vi "Main.vi"() -> ()   [LabVIEW 2017]
uses:
  stateCtrl.ctl
  <vilib>/vision/driver/IMAQdx.llb/IMAQdx Camera Control Mode.ctl
  <resource>/objmgr/imaqdx.rc
  <vilib>/userdefined/High Color/IMAQdx.ctl
panel:
  out "Actual Exposure Time":dbl
  in  "Halt measurement":bool
  in  "Reset spatial\nfreqs":bool
  in  "Run":bool
  in  "stop":bool
  out "Last measurement":timestamp
  out "Measurement in progress":bool
  in  "Measurement interval (s)":dbl
  in  "Number of measurements":dbl=1.0
  in  "Current Measurement number":dbl
  in  "sampleName":string
  in  "savePath":path=path "C:/Users/Roblyer-Admin/Documents/openSFDI/Data"
  out "Current Image Index":i16
  in  "Delay":u32=200
  out "Total Images/wv":dbl
  out "numProfilometry_Images/wv":i32
  out "NumSFDI_images/wv":i32
  out "ImageMatrix":u8[][][](array[numeric])
  in  "Manual\nControl":bool
  out "Colormap":u32[](array[numeric])
  out "Arduino Session":refnum<visa-resource-name>
  in  "error":errorcluster
  out "Camera Session":T1 caption="Session Out"
  out "LED state":bool[](array[boolean])
  in  "Arduino Port":refnum<visa-resource-name>
  out "Image Array":T2[](array[plugin-control])
  in  "Prof. Spatial \nFreq (cycs)":dbl[](array[numeric])
  in  "SFDI Spatial \nFreq (cycs)":dbl[](array[numeric])
  in  "Camera Name":refnum<k21> caption="IMAQdx Session"
  in  "LED\nManual Control":enum16{"Off", "660 nm", "735 nm", "850 nm"}(ring)
  in  "Profilometry Wavelength":enum16{"None", "660 nm", "735 nm", "850 nm"}(ring)=enum."660 nm"
  in  "Dark?":bool
  in  "SFDI?":bool
  in  "Profilometry?":bool
  in  "Exposure Times (ms)":dbl[](array[numeric])=[100.0, 100.0, 100.0, 100.0]
  in  "SFDI wavelengths to use":bool[](array[boolean])
  # "660"
  # "735"
  # "850"
  # "730"
  # "865"
  # "970"
  # "660"
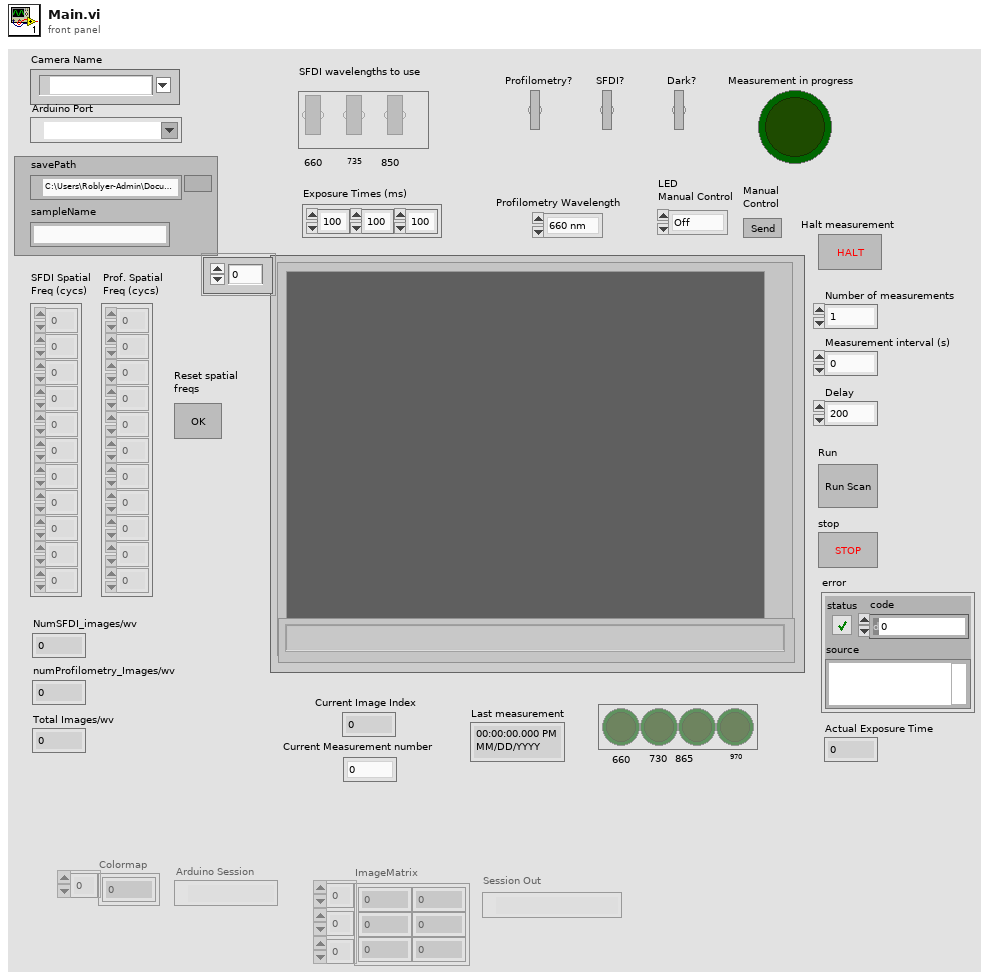
[diagram p1: front panel]
types:
  T1 = typedef "IMAQdx.ctl" = refnum<k21>
  T2 = typedef "IMAQ Image.ctl" = refnum<image>
  T3 = typedef "stateCtrl.ctl" = enum16{"Init", "Wait", "Setup Scan", "Setup Camera", "Run Scan", "Run Profilometry", "Save", "Shutdown", "Run Dark"}
  T4 = enum32{"Invalid", "Standard", "Closed", "Hidden", "Minimized", "Maximized"}
  T5 = typedef "NI_Vision_Acquisition_Software.lvlib/IMAQdx Camera Control Mode.ctl" = enum32{"Controller", "Listener"}
  T6 = cluster{"Left":i32, "Top":i32, "Right":i32, "Bottom":i32}
  T7 = typedef "Image Type" = u32
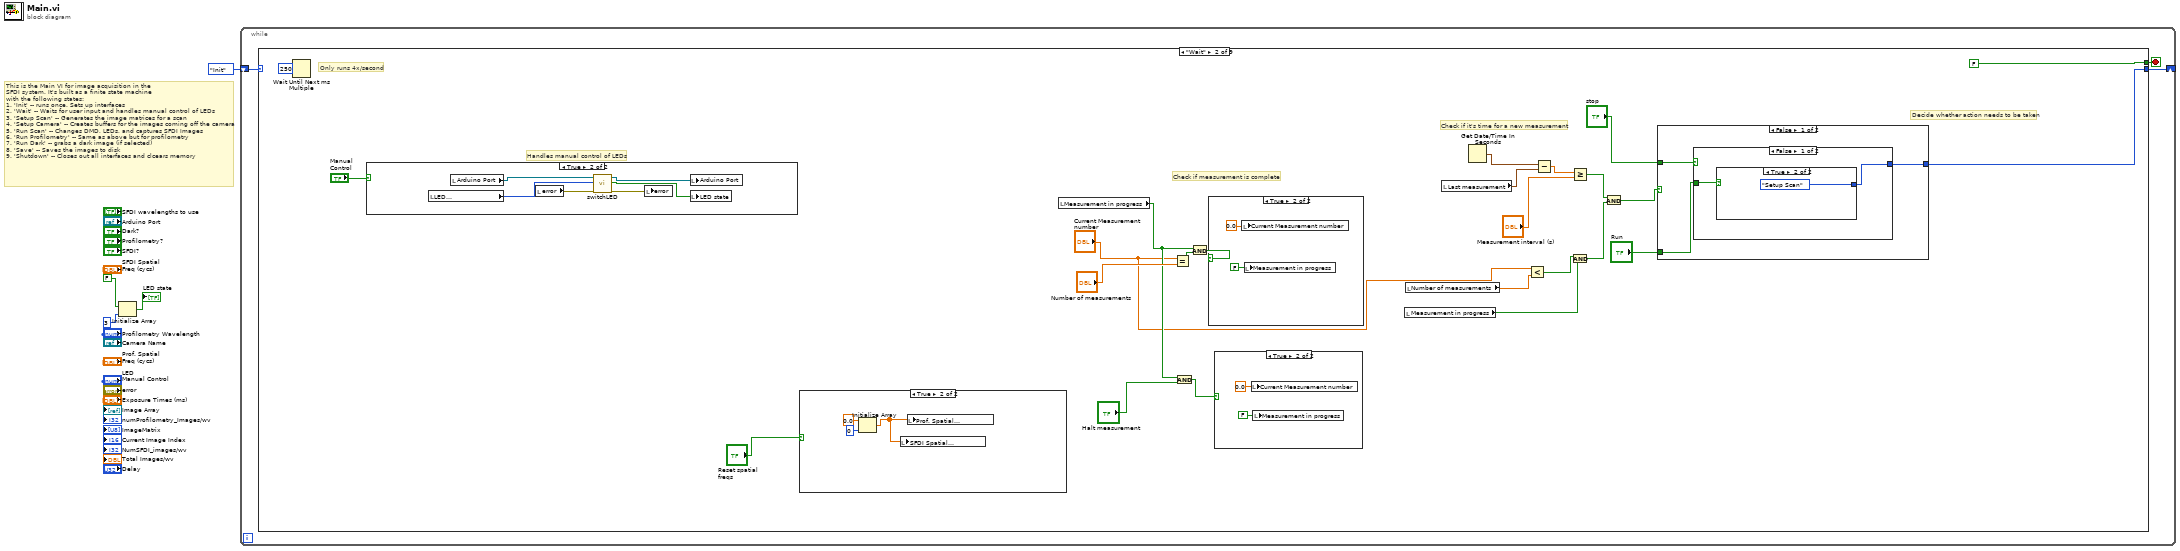
[diagram p0: block diagram]
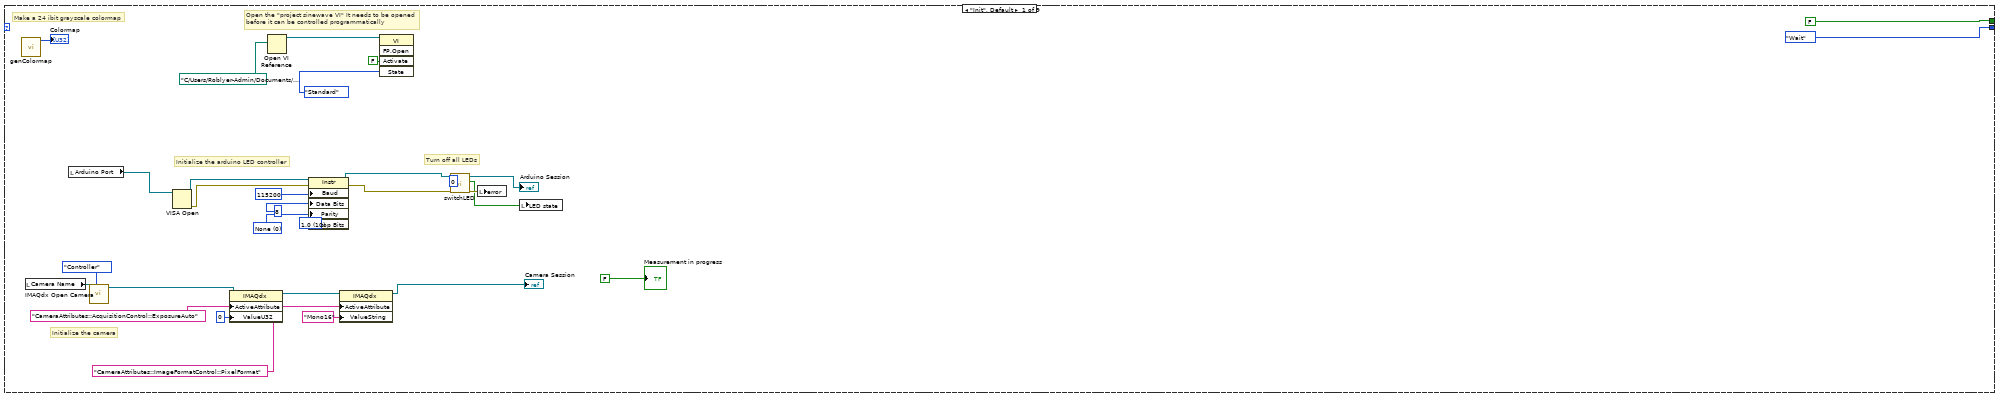
[diagram p2: hidden frame]
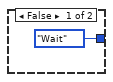
[diagram p5: hidden frame]
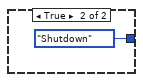
[diagram p6: hidden frame]
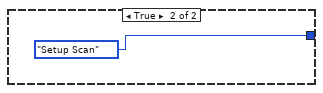
[diagram p7: hidden frame]
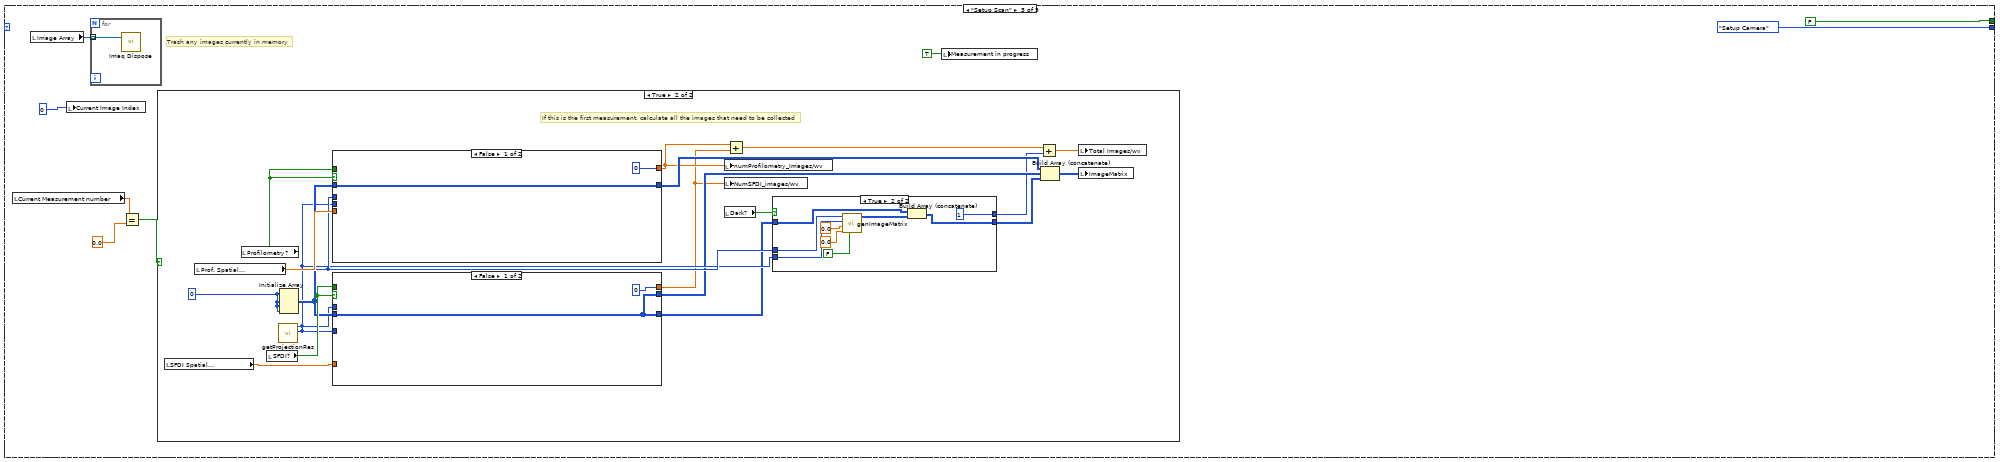
[diagram p10: hidden frame]
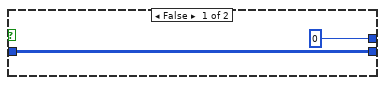
[diagram p12: hidden frame]
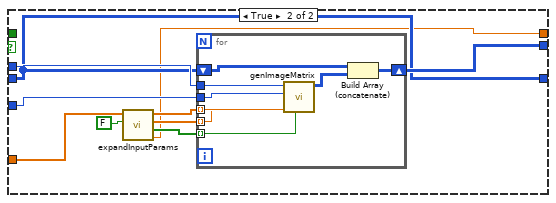
[diagram p13: hidden frame]
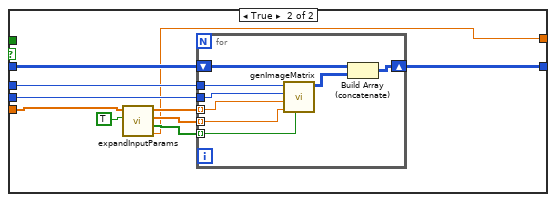
[diagram p14: hidden frame]
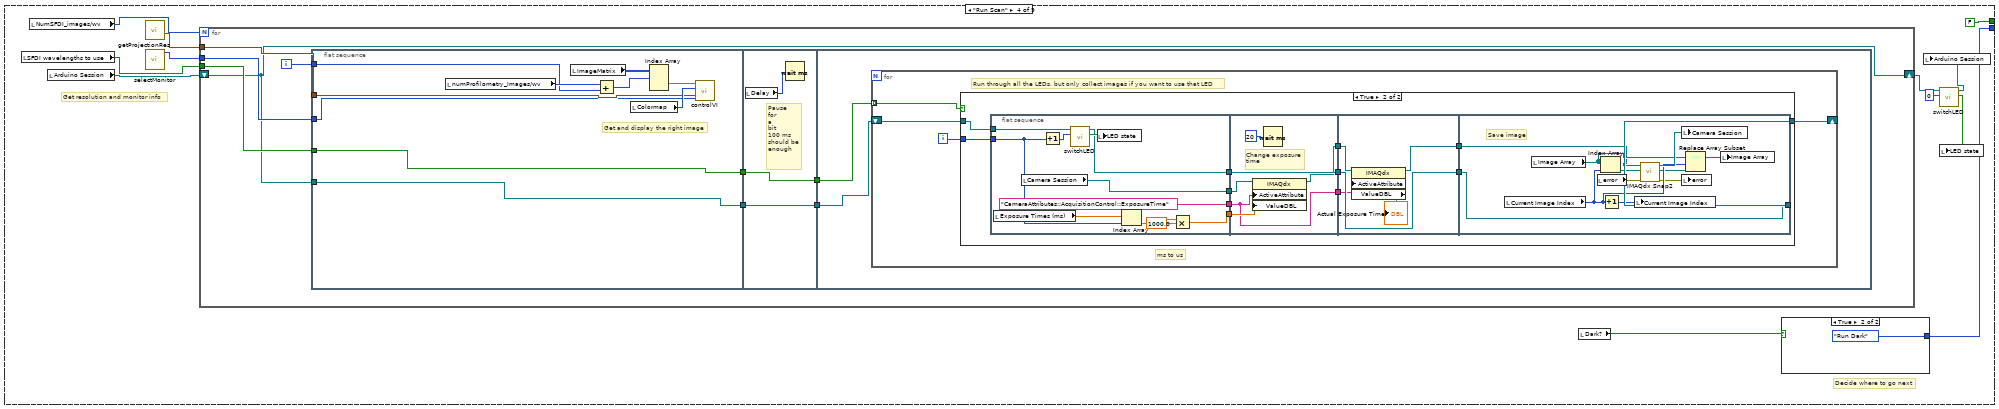
[diagram p15: hidden frame]
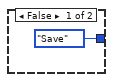
[diagram p16: hidden frame]
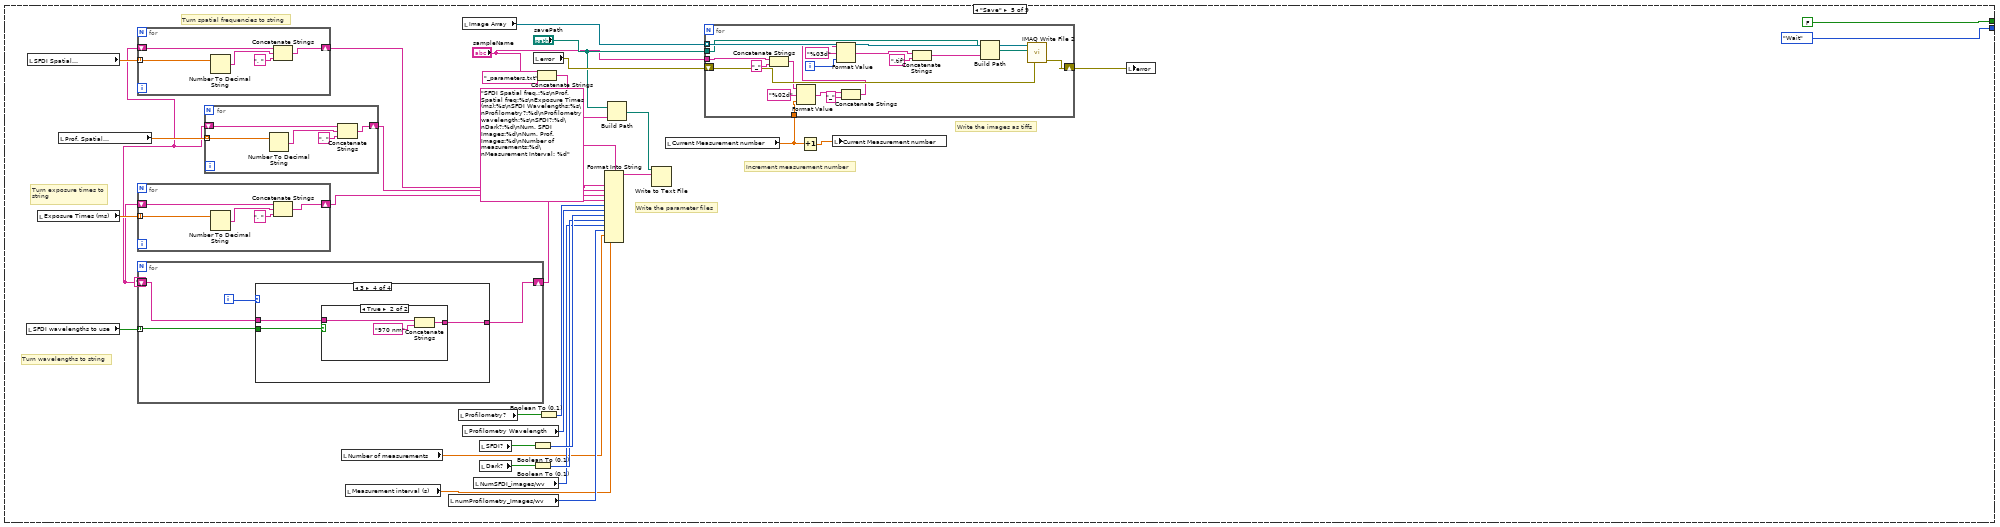
[diagram p18: hidden frame]
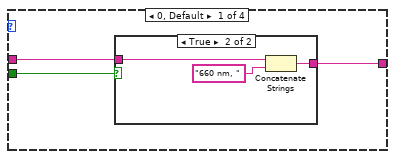
[diagram p19: hidden frame]
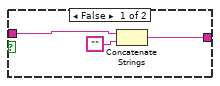
[diagram p20: hidden frame]
diagram:
  # "This is the Main VI for image acquisition in the\nSFDI system. It's built as a finite state machine\nwith the following states:\n1. 'Init' -- runs once. Sets up interfaces\n2. 'Wait' -- Waits for user input and handles manual control of LEDs\n3. 'Setup Scan' -- Generates the image matrices for a scan\n4. 'Setup Camera' -- Creates buffers for the images coming off the camera\n5. 'Run Scan' -- Changes DMD, LEDs, and captures SFDI Images\n6. 'Run Profilometry' -- Same as above but for profilometry\n7. 'Run Dark' -- grabs a dark image (if selected)\n8. 'Save' -- Saves the images to disk\n9. 'Shutdown' -- Closes out all interfaces and clcears memory"
  n1 = Initialize Array(FALSE, 3 ("dimension size")) -> (→"LED state":bool[])
  n2 = while {
    shift-right: [w5] -> _
    shift-left: stateCtrl."Init" -> [w7]
    stop <- w6 stop-if-true
    n3 = case shown="\"Wait\"" w7 {
      tunnel: [stateCtrl."Wait" w60 stateCtrl."Setup Camera" w169 stateCtrl."Wait" stateCtrl."Wait" w372 w425 stateCtrl."Save"] -> w5
      tunnel: [FALSE FALSE FALSE FALSE FALSE TRUE FALSE FALSE FALSE] -> w6
      frame "Init", Default {
        w30 = u16 10 items=["1.0"=10, "1.5"=15, "2.0"=20] ("Serial Settings:Stop Bits")
        w31 = u16 0 items=["None", "Odd", "Even", "Mark", "Space"] ("Serial Settings:Parity")
        # "Turn off all LEDs"
        # "Initialize the arduino LED controller"
        # "Initialize the camera"
        # "Open the \"project sinewave VI\" It needs to be opened \nbefore it can be controlled programmatically"
        # "Make a 24 ibit grayscale colormap"
        n4 = call "genColormap.vi"() -> ("Colormap"=→"Colormap":u32[])  [unwired: 11 in]
        n5 = local read "Camera Name"() -> (w37:refnum<k21>)
        n6 = local read "Arduino Port"() -> (w35:refnum<visa-resource-name>)
        n7 = call <vilib>:"IMAQdx Open Camera.vi"("Camera Control Mode"=IMAQdx_Camera_Control_Mode."Controller", "Session In"=w37) -> ("Session Out"=w14:T1)  [unwired: 1 in, 8 out]
        n8 = VISA Open(VISA resource name=w35) -> (VISA resource name=w34:refnum<visa-resource-name>, error out=w29:errorcluster)  [unwired: 4 in]
        n9 = property class="IMAQdx"(reference=w14, "ActiveAttribute"="CameraAttributes::AcquisitionControl::ExposureAuto", "ValueU32"=u32 0) -> (reference out=w11:T1)  [unwired: 1 in, 1 out]
        n10 = Open VI Reference(vi path=path "C:/Users/Roblyer-Admin/Documents/openSFDI/openSFDI_software/projectSinewave.vi") -> (vi reference=w27:refnum<vi>)  [unwired: 5 in, 1 out]
        n11 = property class="Instr"(reference=w34, error in=w29, "Baud"=u32 115200 ("Serial Settings:Baud Rate"), "Data Bits"=u16 8 ("Serial Settings:Data Bits"), "Parity"=w31, "Stop Bits"=w30) -> (reference out=w23:refnum<visa-resource-name>, error out=w21:errorcluster)
        n12 = property class="IMAQdx"(reference=w11, "ActiveAttribute"="CameraAttributes::ImageFormatControl::PixelFormat", "ValueString"="Mono16") -> (reference out=→"Camera Session":T1)  [unwired: 1 in, 1 out]
        n13 = invoke class="VI" method="FP.Open"(reference=w27, "Activate"=FALSE ("Activate?"), "State"=T4."Standard") -> ()  [unwired: 2 in, 5 out]
        n14 = call "switchLED.vi"("error in (no error)"=w21, "Which LED"=u8 0, "Arduino session"=w23) -> ("error out"=w19:errorcluster, "LED vector"=w17:bool[], "Arduino session"=→"Arduino Session":refnum<visa-resource-name>)  [unwired: 6 in]
        n15 = local write "error"(w19) -> ()
        n16 = local write "LED state"(w17) -> ()
        "Measurement in progress" <- FALSE ("Measurement in progress")
      }
      frame "Wait" {
        # "Decide whether action needs to be taken"
        # "Check if it's time for a new measurement"
        # "Check if measurement is complete"
        # "Handles manual control of LEDs"
        # "Only runs 4x/second"
        n17 = Wait Until Next ms Multiple(millisecond multiple=u32 250 ("milliseconds to wait")) -> ()  [unwired: 1 out]
        n18 = case shown="True" "Manual\nControl" {
          frame False {
          }
          frame True {
            n19 = local read "LED\nManual Control"() -> (w83:enum16{"Off", "660 nm", "735 nm", "850 nm"})
            n20 = local read "Arduino Port"() -> (w82:refnum<visa-resource-name>)
            n21 = local read "error"() -> (w81:errorcluster)
            n22 = call "switchLED.vi"("error in (no error)"=w81, "Which LED"=w83, "Arduino session"=w82) -> ("error out"=w78:errorcluster, "LED vector"=w80:bool[], "Arduino session"=w79:refnum<visa-resource-name>)  [unwired: 6 in]
            n23 = local write "error"(w78) -> ()
            n24 = local write "Arduino Port"(w79) -> ()
            n25 = local write "LED state"(w80) -> ()
          }
        }
        n26 = case shown="True" "Reset spatial\nfreqs" {
          frame False {
          }
          frame True {
            n27 = Initialize Array(0.0 ("element"), 0 ("dimension size")) -> (w64:dbl[])
            n28 = local write "SFDI Spatial \nFreq (cycs)"(w64) -> ()
            n29 = local write "Prof. Spatial \nFreq (cycs)"(w64) -> ()
          }
        }
        n30 = local read "Measurement in progress"() -> (w41:bool)
        n31 = Equal?(x="Current Measurement number", y="Number of measurements") -> (x = y?=w52:bool)
        n32 = And(x=w41, y="Halt measurement") -> (x .and. y?=w43:bool)
        n33 = And(x=w41, y=w52) -> (x .and. y?=w51:bool)
        n34 = case shown="True" w51 {
          frame False {
          }
          frame True {
            n35 = local write "Current Measurement number"(0.0 ("Current Measurement number")) -> ()
            n36 = local write "Measurement in progress"(FALSE ("Measurement in progress")) -> ()
          }
        }
        n37 = case shown="True" w43 {
          frame False {
          }
          frame True {
            n38 = local write "Current Measurement number"(0.0 ("Current Measurement number")) -> ()
            n39 = local write "Measurement in progress"(FALSE ("Measurement in progress")) -> ()
          }
        }
        n40 = local read "Measurement in progress"() -> (w48:bool)
        n41 = local read "Number of measurements"() -> (w50:dbl)
        n42 = local read "Last measurement"() -> (w56:timestamp)
        n43 = Get Date/Time In Seconds() -> (seconds since 1Jan1904=w57:timestamp)
        n44 = Less?(x="Current Measurement number", y=w50) -> (x < y?=w49:bool)
        n45 = Subtract(x=w57, y=w56) -> (x-y=w55:dbl)
        n46 = Greater Or Equal?(x=w55, y="Measurement interval (s)") -> (x >= y?=w47:bool)
        n47 = And(x=w49, y=w48) -> (x .and. y?=w46:bool)
        n48 = And(x=w47, y=w46) -> (x .and. y?=w45:bool)
        n49 = case shown="False" w45 {
          tunnel: [w69 stateCtrl."Setup Scan"] -> w60
          tunnel: "stop" -> [w68 _]
          tunnel: "Run" -> [w67 _]
          frame False {
            n50 = case shown="False" w68 {
              tunnel: [w70 stateCtrl."Shutdown"] -> w69
              tunnel: w67 -> [w71 _]
              frame False {
                n51 = case shown="True" w71 {
                  tunnel: [stateCtrl."Wait" stateCtrl."Setup Scan"] -> w70
                  frame False {
                  }
                  frame True {
                  }
                }
              }
              frame True {
              }
            }
          }
          frame True {
          }
        }
      }
      frame "Setup Scan" {
        # "Trash any images currently in memory"
        n52 = local read "Current Measurement number"() -> (w87:dbl)
        n53 = local read "Image Array"() -> (w88:T2[])
        n54 = local write "Current Image Index"(i16 0 ("Current Image Index")) -> ()
        n55 = for {
          tunnel: w88 -> [w162] mode=indexing
          n56 = call "Imaq Dispose"("Image"=w162) -> ()  [unwired: 5 in, 1 out]
        }
        n57 = Equal?(x=w87, y=0.0) -> (x = y?=w85:bool)
        n58 = case shown="True" w85 {
          frame False {
          }
          frame True {
            w105 = 0
            # "If this is the first measurement, calculate all the images that need to be collected"
            n59 = local read "SFDI Spatial \nFreq (cycs)"() -> (w106:dbl[])
            n60 = local read "Prof. Spatial \nFreq (cycs)"() -> (w108:dbl[])
            n61 = local read "Profilometry?"() -> (w109:bool)
            n62 = local read "SFDI?"() -> (w107:bool)
            n63 = call "getProjectionRes.vi"() -> ("YRes"=w102:i32, "XRes"=w103:i32)  [unwired: 9 in, 1 out]
            n64 = Initialize Array(w105, w105, w105, w105) -> (w104:i32[][][])
            n65 = case shown="False" w109 {
              tunnel: w103 -> [_ w150]
              tunnel: w102 -> [_ w149]
              tunnel: w109 -> [_ _]
              tunnel: w108 -> [_ w148]
              tunnel: w104 -> [w143 w147]
              tunnel: [w143 w145] -> w101
              tunnel: [0 w144] -> w96
              frame False {
              }
              frame True {
                n66 = call "expandInputParams.vi"("Profilometry?"=TRUE, "Frequencies"=w148) -> ("Number Images"=w144:dbl, "Orientation Vector"=w153:bool[], "Phase Vector"=w152:dbl[], "Frequency Vector"=w151:dbl[])  [unwired: 6 in]
                n67 = for {
                  tunnel: w153 -> [w161] mode=indexing
                  tunnel: w152 -> [w160] mode=indexing
                  tunnel: w151 -> [w159] mode=indexing
                  tunnel: w150 -> [w158]
                  tunnel: w149 -> [w157]
                  shift-right: [w155] -> w145
                  shift-left: w147 -> [w154]
                  n68 = call "genImageMatrix.vi"("Orientation"=w161, "Phase"=w160, "Cycles"=w159, "Y resolution"=w157, "X Resolution"=w158) -> ("Scan Image"=w156:u8[][])  [unwired: 5 in, 1 out]
                  n69 = Build Array (concatenate)(w154, w156) -> (w155:i32[][][])
                }
              }
            }
            n70 = case shown="False" w107 {
              tunnel: w107 -> [_ _]
              tunnel: w106 -> [_ w133]
              tunnel: w104 -> [w123 w125]
              tunnel: w103 -> [_ w131]
              tunnel: w102 -> [_ w130]
              tunnel: [w123 w126] -> w100
              tunnel: [w123 w125] -> w98
              tunnel: [0 w124] -> w95
              frame False {
              }
              frame True {
                n71 = call "expandInputParams.vi"("Profilometry?"=FALSE, "Frequencies"=w133) -> ("Number Images"=w124:dbl, "Orientation Vector"=w127:bool[], "Phase Vector"=w128:dbl[], "Frequency Vector"=w129:dbl[])  [unwired: 6 in]
                n72 = for {
                  shift-right: [w140] -> w126
                  shift-left: w125 -> [w139]
                  tunnel: w131 -> [w138]
                  tunnel: w130 -> [w137]
                  tunnel: w129 -> [w136] mode=indexing
                  tunnel: w128 -> [w135] mode=indexing
                  tunnel: w127 -> [w134] mode=indexing
                  n73 = call "genImageMatrix.vi"("Orientation"=w134, "Phase"=w135, "Cycles"=w136, "Y resolution"=w137, "X Resolution"=w138) -> ("Scan Image"=w141:u8[][])  [unwired: 5 in, 1 out]
                  n74 = Build Array (concatenate)(w139, w141) -> (w140:i32[][][])
                }
              }
            }
            n75 = local write "numProfilometry_Images/wv"(w96) -> ()
            n76 = local write "NumSFDI_images/wv"(w95) -> ()
            n77 = local read "Dark?"() -> (w110:bool)
            n78 = Add(x=w96, y=w95) -> (x+y=w94:dbl)
            n79 = case shown="True" w110 {
              tunnel: w103 -> [_ w121]
              tunnel: w102 -> [_ w120]
              tunnel: [w112 w114] -> w99
              tunnel: w98 -> [w112 w116]
              tunnel: [0 1] -> w93
              frame False {
              }
              frame True {
                n80 = call "genImageMatrix.vi"("Orientation"=FALSE, "Phase"=0.0, "Cycles"=0.0, "Y resolution"=w120, "X Resolution"=w121) -> ("Scan Image"=w115:u8[][])  [unwired: 5 in, 1 out]
                n81 = Build Array (concatenate)(w116, w115) -> (w114:i32[][][])
              }
            }
            n82 = Add(x=w94, y=w93) -> (x+y=w92:dbl)
            n83 = Build Array (concatenate)(w101, w100, w99) -> (w97:i32[][][])
            n84 = local write "Total Images/wv"(w92) -> ()
            n85 = local write "ImageMatrix"(w97) -> ()
          }
        }
        n86 = local write "Measurement in progress"(TRUE) -> ()
      }
      frame "Run Scan" {
        # "Decide where to go next"
        # "Get resolution and monitor info"
        n87 = local read "SFDI wavelengths to use"() -> (w170:bool[])
        n88 = local read "NumSFDI_images/wv"() -> (w168:i32)
        n89 = local read "Arduino Session"() -> (w171:refnum<visa-resource-name>)
        n90 = call "getProjectionRes.vi"() -> ("projBounds"=w173:T6)  [unwired: 9 in, 2 out]
        n91 = call "selectMonitor.vi"() -> ("monitor to use"=w172:i32)  [unwired: 11 in]
        n92 = for {
          N: w168 -> [_]
          tunnel: w173 -> [w184]
          tunnel: w172 -> [w183]
          tunnel: w170 -> [w180]
          shift-right: [w177] -> w166
          shift-left: w171 -> [w177]
          i -> [w185]
          n93 = flat-sequence {
            tunnel: w185 -> [w194]
            tunnel: w184 -> [w189]
            tunnel: w183 -> [w188]
            tunnel: [w187] -> w181
            tunnel: w180 -> [w187]
            tunnel: [w186] -> w178
            tunnel: w177 -> [w186]
            tunnel: [w198] -> w182
            tunnel: w181 -> [w198]
            tunnel: [w197] -> w179
            tunnel: w178 -> [w197]
            tunnel: w182 -> [w200]
            tunnel: w179 -> [w199]
            frame #0 {
              # "Get and display the right image"
              n94 = local read "numProfilometry_Images/wv"() -> (w195:i32)
              n95 = local read "ImageMatrix"() -> (w193:u8[][][])
              n96 = Add(x=w195, y=w194) -> (x+y=w192:i32)
              n97 = local read "Colormap"() -> (w190:u32[])
              n98 = Index Array(array=w193, index (dim 0)=w192) -> (element=w191:u8[][])  [unwired: 2 in]
              n99 = call "controlVI.vi"("monitorToUse"=w188, "Front Panel Window:Window Bounds"=w189, "colors"=w190, "8-bit pixmap"=w191) -> ()  [unwired: 7 in, 1 out]
            }
            frame #1 {
              # "Pause\nfor\na\nbit\n100 ms\nshould be\nenough"
              n100 = local read "Delay"() -> (w196:u32)
              n101 = Wait (ms)(milliseconds to wait=w196) -> ()  [unwired: 1 out]
            }
            frame #2 {
              n102 = for {
                shift-right: [w202] -> _
                shift-left: w199 -> [w203]
                tunnel: w200 -> [w201] mode=indexing
                i -> [w204]
                # "ms to us"
                # "Run through all the LEDs, but only collect images if you want to use that LED"
                n103 = case shown="True" w201 {
                  tunnel: w204 -> [_ w217]
                  tunnel: w203 -> [w205 w216]
                  tunnel: [w205 w215] -> w202
                  frame False {
                  }
                  frame True {
                    n104 = flat-sequence {
                      tunnel: w217 -> [w221]
                      tunnel: w216 -> [w227]
                      tunnel: [w225] -> w214
                      tunnel: [w224] -> w213
                      tunnel: ["CameraAttributes::AcquisitionControl::ExposureTime"] -> w212
                      tunnel: [w218] -> w211
                      tunnel: [w233] -> w210
                      tunnel: w214 -> [w233]
                      tunnel: [w231] -> w208
                      tunnel: w213 -> [w232]
                      tunnel: w212 -> [w229]
                      tunnel: w211 -> [w230]
                      tunnel: [w229] -> w206
                      tunnel: w210 -> [w237]
                      tunnel: [w237] -> w209
                      tunnel: w208 -> [w239]
                      tunnel: [w238] -> w207
                      tunnel: w206 -> [w235]
                      tunnel: [w243] -> w215
                      tunnel: w209 -> [w243]
                      tunnel: w207 -> [w240]
                      frame #0 {
                        n105 = local read "Exposure Times (ms)"() -> (w222:dbl[])
                        n106 = local read "Camera Session"() -> (w224:T1)
                        n107 = Increment(x=w221) -> (x+1=w228:i32)
                        n108 = call "switchLED.vi"("Which LED"=w228, "Arduino session"=w227) -> ("LED vector"=w226:bool[], "Arduino session"=w225:refnum<visa-resource-name>)  [unwired: 7 in, 1 out]
                        n109 = local write "LED state"(w226) -> ()
                        n110 = Index Array(array=w222, index=w221) -> (element=w220:dbl)
                        n111 = Multiply(x=w220, y=1000.0) -> (x*y=w218:dbl)
                      }
                      frame #1 {
                        # "Change exposure\ntime"
                        n112 = property class="IMAQdx"(reference=w232, "ActiveAttribute"=w229, "ValueDBL"=w230) -> (reference out=w231:T1)  [unwired: 1 in, 1 out]
                        n113 = Wait (ms)(milliseconds to wait=u32 20) -> ()  [unwired: 1 out]
                      }
                      frame #2 {
                        n114 = property class="IMAQdx"(reference=w239, "ActiveAttribute"=w235) -> (reference out=w238:T1, "ValueDBL"=→"Actual Exposure Time")  [unwired: 1 in, 1 out]
                      }
                      frame #3 {
                        # "Save image"
                        n115 = local read "Current Image Index"() -> (w246:i16)
                        n116 = local read "Image Array"() -> (w247:T2[])
                        n117 = local read "error"() -> (w242:errorcluster)
                        n118 = Index Array(array=w247, index=w246) -> (element=w249:T2)
                        n119 = Increment(x=w246) -> (x+1=w248:i16)
                        n120 = local write "Current Image Index"(w248) -> ()
                        n121 = call <vilib>:"IMAQdx Snap2.vi"("error in"=w242, "Image In"=w249, "Session In"=w240) -> ("error out"=w241:errorcluster, "Image Out"=w245:T2, "Session Out"=w250:T1)  [unwired: 6 in]
                        n122 = local write "Camera Session"(w250) -> ()
                        n123 = local write "error"(w241) -> ()
                        n124 = Replace Array Subset(array=w247, new element=w245, index=w246) -> (w244:T2[])
                        n125 = local write "Image Array"(w244) -> ()
                      }
                    }
                  }
                }
              }
            }
          }
        }
        n126 = local read "Dark?"() -> (w167:bool)
        n127 = case shown="True" w167 {
          tunnel: [stateCtrl."Save" stateCtrl."Run Dark"] -> w169
          frame False {
          }
          frame True {
          }
        }
        n128 = call "switchLED.vi"("Which LED"=u8 0, "Arduino session"=w166) -> ("LED vector"=w164:bool[], "Arduino session"=w163:refnum<visa-resource-name>)  [unwired: 7 in, 1 out]
        n129 = local write "Arduino Session"(w163) -> ()
        n130 = local write "LED state"(w164) -> ()
      }
      frame "Save" {
        w257 = ""
        # "Increment measurement number"
        # "Write the images as tiffs"
        # "Write the parameter files"
        # "Turn wavelengths to string"
        # "Turn exposure times to\nstring"
        # "Turn spatial frequencies to string"
        n131 = local read "SFDI wavelengths to use"() -> (w255:bool[])
        n132 = local read "SFDI Spatial \nFreq (cycs)"() -> (w276:dbl[])
        n133 = local read "Exposure Times (ms)"() -> (w274:dbl[])
        n134 = local read "Prof. Spatial \nFreq (cycs)"() -> (w275:dbl[])
        n135 = for {
          tunnel: w276 -> [w339] mode=indexing
          shift-right: [w336] -> w273
          shift-left: w257 -> [w335]
          n136 = Number To Decimal String(number=w339) -> (decimal integer string=w337:string)  [unwired: 1 in]
          n137 = Concatenate Strings(w335, w337, ", ") -> (w336:string)
        }
        n138 = for {
          tunnel: w274 -> [w329] mode=indexing
          shift-right: [w326] -> w271
          shift-left: w257 -> [w325]
          n139 = Number To Decimal String(number=w329) -> (decimal integer string=w327:string)  [unwired: 1 in]
          n140 = Concatenate Strings(w325, w327, ", ") -> (w326:string)
        }
        n141 = for {
          shift-right: [w286] -> w270
          shift-left: w257 -> [w285]
          tunnel: w255 -> [w287] mode=indexing
          i -> [w288]
          n142 = case shown="3" w288 {
            tunnel: w287 -> [w291 w300 w309 w318]
            tunnel: [w290 w299 w308 w316] -> w286
            tunnel: w285 -> [w289 w298 w307 w317]
            frame 0, Default {
              n143 = case shown="True" w291 {
                tunnel: [w294 w295] -> w290
                tunnel: w289 -> [w293 w297]
                frame False {
                  n144 = Concatenate Strings(w293, "") -> (w294:string)
                }
                frame True {
                  n145 = Concatenate Strings(w297, "660 nm, ") -> (w295:string)
                }
              }
            }
            frame 1 {
              n146 = case shown="True" w300 {
                tunnel: [w301 w304] -> w299
                tunnel: w298 -> [w303 w306]
                frame False {
                  n147 = Concatenate Strings(w303, "") -> (w301:string)
                }
                frame True {
                  n148 = Concatenate Strings(w306, "730 nm, ") -> (w304:string)
                }
              }
            }
            frame 2 {
              n149 = case shown="True" w309 {
                tunnel: [w310 w313] -> w308
                tunnel: w307 -> [w312 w314]
                frame False {
                  n150 = Concatenate Strings(w312, "") -> (w310:string)
                }
                frame True {
                  n151 = Concatenate Strings(w314, "865 nm, ") -> (w313:string)
                }
              }
            }
            frame 3 {
              n152 = case shown="True" w318 {
                tunnel: w317 -> [w321 w324]
                tunnel: [w319 w322] -> w316
                frame False {
                  n153 = Concatenate Strings(w321, "") -> (w319:string)
                }
                frame True {
                  n154 = Concatenate Strings(w324, "970 nm") -> (w322:string)
                }
              }
            }
          }
        }
        n155 = for {
          tunnel: w275 -> [w334] mode=indexing
          shift-right: [w331] -> w272
          shift-left: w257 -> [w330]
          n156 = Number To Decimal String(number=w334) -> (decimal integer string=w332:string)  [unwired: 1 in]
          n157 = Concatenate Strings(w330, w332, ", ") -> (w331:string)
        }
        n158 = local read "Number of measurements"() -> (w252:dbl)
        n159 = local read "Measurement interval (s)"() -> (w251:dbl)
        n160 = local read "numProfilometry_Images/wv"() -> (w259:i32)
        n161 = local read "Profilometry?"() -> (w277:bool)
        n162 = local read "Image Array"() -> (w282:T2[])
        n163 = local read "Profilometry Wavelength"() -> (w256:enum16{"None", "660 nm", "735 nm", "850 nm"})
        n164 = local read "NumSFDI_images/wv"() -> (w260:i32)
        n165 = local read "SFDI?"() -> (w278:bool)
        n166 = local read "Dark?"() -> (w279:bool)
        n167 = Boolean To (0,1)(Boolean=w278) -> (0, 1=w268:i16)
        n168 = Boolean To (0,1)(Boolean=w279) -> (0, 1=w267:i16)
        n169 = local read "error"() -> (w281:errorcluster)
        n170 = Concatenate Strings("sampleName", "_parameters.txt" ("string")) -> (w263:string)
        n171 = Boolean To (0,1)(Boolean=w277) -> (0, 1=w269:i16)
        n172 = Format Into String(format string="SFDI Spatial freq.:%s\nProf. Spatial freq:%s\nExposure Times (ms):%s\nSFDI Wavelengths:%s\nProfilometry?:%d\nProfilometry wavelength:%s\nSFDI?:%d\nDark?:%d\nNum. SFDI Images:%d\nNum. Prof. Images:%d\nNumber of measurements:%d\nMeasurement Interval: %d", w273, w272, w271, w270, w269, w256, w268, w267, w260, w259, w252, w251) -> (resulting string=w261:string)  [unwired: 2 in, 1 out]
        n173 = Build Path(base path="savePath", name or relative path=w263) -> (appended path=w262:path)
        n174 = Write to Text File(file (use dialog)=w262, text=w261) -> ()  [unwired: 2 in, 3 out]
        n175 = local read "Current Measurement number"() -> (w253:dbl)
        n176 = for {
          tunnel: w282 -> [w357] mode=indexing
          shift-right: [w346] -> w280
          shift-left: w281 -> [w356]
          tunnel: "savePath" -> [w355]
          tunnel: "sampleName" -> [w347]
          tunnel: w253 -> [w344]
          i -> [w352]
          n177 = Concatenate Strings(w347, "_") -> (w343:string)
          n178 = Format Value(string ("")=w343, format string="%02d", value (0)=w344) -> (output string=w342:string)
          n179 = Concatenate Strings(w342, "_" ("string")) -> (w340:string)
          n180 = Format Value(string ("")=w340, format string="%03d", value (0)=w352) -> (output string=w351:string)
          n181 = Concatenate Strings(w351, ".tif" ("string")) -> (w349:string)
          n182 = Build Path(base path=w355, name or relative path=w349) -> (appended path=w348:path)
          n183 = call-poly "IMAQ Write File 2"("error in (no error)"=w356, "File Path"=w348, "Image"=w357) -> ("error out"=w346:errorcluster)  [unwired: 7 in, 1 out]
        }
        n184 = Increment(x=w253) -> (x+1=w254:dbl)
        n185 = local write "Current Measurement number"(w254) -> ()
        n186 = local write "error"(w280) -> ()
      }
      frame "Shutdown" {
        # "Stop the while loop"
        # "Turn off and close session with Arduino"
        # "Close camera"
        # "Clean up memory"
        n187 = local read "Image Array"() -> (w358:T2[])
        n188 = local read "Camera Session"() -> (w363:T1)
        n189 = for {
          tunnel: w358 -> [w368] mode=indexing
          n190 = call "Imaq Dispose"("Image"=w368) -> ()  [unwired: 5 in, 1 out]
        }
        n191 = local read "error"() -> (w362:errorcluster)
        n192 = local read "Arduino Session"() -> (w365:refnum<visa-resource-name>)
        n193 = call <vilib>:"IMAQdx Close Camera.vi"("error in"=w362, "Session In"=w363) -> ("error out"=w361:errorcluster)  [unwired: 9 out]
        n194 = call "switchLED.vi"("error in (no error)"=w361, "Which LED"=u8 0, "Arduino session"=w365) -> ("error out"=w360:errorcluster, "Arduino session"=w364:refnum<visa-resource-name>)  [unwired: 6 in, 1 out]
        n195 = VISA Close(VISA resource name=w364, error in (no error)=w360) -> ()  [unwired: 1 out]
      }
      frame "Run Profilometry" {
        # "Decide whether Dark, or SFDI needs to be done"
        # "Turn off LEDs when done"
        # "Turn on LED"
        # "Profilometry always comes before SFDI or Dark\nmeasurements"
        n196 = local read "Profilometry Wavelength"() -> (w384:enum16{"None", "660 nm", "735 nm", "850 nm"})
        n197 = local read "Arduino Session"() -> (w383:refnum<visa-resource-name>)
        n198 = local read "numProfilometry_Images/wv"() -> (w370:i32)
        n199 = local read "error"() -> (w382:errorcluster)
        n200 = call "switchLED.vi"("error in (no error)"=w382, "Which LED"=w384, "Arduino session"=w383) -> ("error out"=w377:errorcluster, "LED vector"=w381:bool[], "Arduino session"=w379:refnum<visa-resource-name>)  [unwired: 6 in]
        n201 = local write "LED state"(w381) -> ()
        n202 = for {
          N: w370 -> [_]
          shift-right: [w391] -> w378
          shift-left: w377 -> [w390]
          i -> [w394]
          # "Take an image for each profilometry pattern selected"
          n203 = flat-sequence {
            tunnel: w394 -> [w400]
            tunnel: [w395] -> w392
            tunnel: w390 -> [w395]
            tunnel: [w402] -> w393
            tunnel: w392 -> [w402]
            tunnel: w393 -> [w411]
            tunnel: [w407] -> w391
            frame #0 {
              # "Project pattern"
              n204 = local read "ImageMatrix"() -> (w401:u8[][][])
              n205 = local read "Colormap"() -> (w399:u32[])
              n206 = Index Array(array=w401, index (dim 0)=w400) -> (element=w398:u8[][])  [unwired: 2 in]
              n207 = call "getProjectionRes.vi"() -> ("projBounds"=w397:T6)  [unwired: 9 in, 2 out]
              n208 = call "selectMonitor.vi"() -> ("monitor to use"=w396:i32)  [unwired: 11 in]
              n209 = call "controlVI.vi"("monitorToUse"=w396, "Front Panel Window:Window Bounds"=w397, "colors"=w399, "8-bit pixmap"=w398) -> ()  [unwired: 7 in, 1 out]
            }
            frame #1 {
              n210 = local read "Delay"() -> (w403:u32)
              n211 = Wait (ms)(milliseconds to wait=w403) -> ()  [unwired: 1 out]
            }
            frame #2 {
              n212 = local read "Current Image Index"() -> (w405:i16)
              n213 = local read "Image Array"() -> (w409:T2[])
              n214 = local read "Camera Session"() -> (w413:T1)
              n215 = Increment(x=w405) -> (x+1=w406:i16)
              n216 = Index Array(array=w409, index=w405) -> (element=w412:T2)
              n217 = local write "Current Image Index"(w406) -> ()
              n218 = call <vilib>:"IMAQdx Snap2.vi"("error in"=w411, "Image In"=w412, "Session In"=w413) -> ("error out"=w407:errorcluster, "Image Out"=w410:T2, "Session Out"=w404:T1)  [unwired: 6 in]
              n219 = Replace Array Subset(array=w409, new element=w410, index=w405) -> (w408:T2[])
              n220 = local write "Camera Session"(w404) -> ()
              n221 = local write "Image Array"(w408) -> ()
            }
          }
        }
        n222 = call "switchLED.vi"("error in (no error)"=w378, "Which LED"=u8 0, "Arduino session"=w379) -> ("error out"=w375:errorcluster, "LED vector"=w376:bool[], "Arduino session"=w374:refnum<visa-resource-name>)  [unwired: 6 in]
        n223 = local write "error"(w375) -> ()
        n224 = local write "Arduino Session"(w374) -> ()
        n225 = local write "LED state"(w376) -> ()
        n226 = local read "SFDI?"() -> (w373:bool)
        n227 = local read "Dark?"() -> (w369:bool)
        n228 = case shown="False" w373 {
          tunnel: [w385 stateCtrl."Run Scan"] -> w372
          tunnel: w369 -> [w386 _]
          frame False {
            n229 = case shown="False" w386 {
              tunnel: [stateCtrl."Save" stateCtrl."Run Dark"] -> w385
              frame False {
              }
              frame True {
              }
            }
          }
          frame True {
          }
        }
      }
      frame "Setup Camera" {
        # "Decide where to go next"
        # "Save start time"
        # "Calculate total number of images to collect"
        # "Do camera stuff here"
        n230 = local read "SFDI wavelengths to use"() -> (w424:bool[])
        n231 = Boolean To (0,1)(Boolean=w424) -> (0, 1=w423:i16[])
        n232 = local read "NumSFDI_images/wv"() -> (w421:i32)
        n233 = local read "numProfilometry_Images/wv"() -> (w419:i32)
        n234 = Add Array Elements(numeric array=w423) -> (sum=w422:i16)
        n235 = Multiply(x=w422, y=w421) -> (x*y=w420:i32)
        n236 = Add(x=w420, y=w419) -> (x+y=w416:i32)
        n237 = local read "Dark?"() -> (w417:bool)
        n238 = case shown="False" w417 {
          tunnel: w416 -> [w430 w432]
          tunnel: [w430 w431] -> w415
          frame False {
          }
          frame True {
            n239 = Increment(x=w432) -> (x+1=w431:i32)
          }
        }
        n240 = local read "error"() -> (w429:errorcluster)
        n241 = for {
          N: w415 -> [_]
          tunnel: w429 -> [w448]
          tunnel: [w447] -> w427 mode=indexing
          tunnel: [w446] -> w428
          i -> [w445]
          w442 = T7 7 items=["Grayscale (U8)", "Grayscale (I16)", "Grayscale (SGL)", "Complex (CSG)", "RGB (U32)", "HSL (U32)", "RGB (U64)", "Grayscale (U16)"] ("Image Type")
          # "Reserve memory for images"
          n242 = Format Into String(format string="image%d" ("Image Name"), w445) -> (resulting string=w444:string)  [unwired: 2 in, 1 out]
          n243 = call "IMAQ Create"("Image Name"=w444, "Image Type"=w442, "error in (no error)"=w448) -> ("New Image"=w447:T2, "error out"=w446:errorcluster)  [unwired: 1 in, 1 out]
        }
        n244 = Get Date/Time In Seconds() -> (seconds since 1Jan1904=→"Last measurement":timestamp)
        n245 = local write "error"(w428) -> ()
        n246 = local write "Image Array"(w427) -> ()
        n247 = local read "Profilometry?"() -> (w426:bool)
        n248 = case shown="False" w426 {
          tunnel: [w434 stateCtrl."Run Profilometry"] -> w425
          frame False {
            n249 = local read "SFDI?"() -> (w435:bool)
            n250 = local read "Dark?"() -> (w433:bool)
            n251 = case shown="False" w435 {
              tunnel: [w436 stateCtrl."Run Scan"] -> w434
              tunnel: w433 -> [w437 _]
              frame False {
                n252 = case shown="True" w437 {
                  tunnel: [stateCtrl."Wait" stateCtrl."Run Dark"] -> w436
                  frame False {
                  }
                  frame True {
                  }
                }
              }
              frame True {
              }
            }
          }
          frame True {
          }
        }
      }
      frame "Run Dark" {
        # "Always save after\ndark measurement"
        # "Dark always comes after SFDI and profilometry"
        n253 = flat-sequence {
          tunnel: [w453] -> w450
          tunnel: [w459] -> w451
          tunnel: w450 -> [w459]
          tunnel: w451 -> [w467]
          frame #0 {
            # "Turn off all LEDs"
            n254 = local read "Arduino Session"() -> (w457:refnum<visa-resource-name>)
            n255 = local read "error"() -> (w454:errorcluster)
            n256 = call "switchLED.vi"("error in (no error)"=w454, "Which LED"=u8 0, "Arduino session"=w457) -> ("error out"=w453:errorcluster, "LED vector"=w455:bool[], "Arduino session"=w456:refnum<visa-resource-name>)  [unwired: 6 in]
            n257 = local write "Arduino Session"(w456) -> ()
            n258 = local write "LED state"(w455) -> ()
          }
          frame #1 {
            n259 = Wait (ms)(milliseconds to wait=u32 10) -> ()  [unwired: 1 out]
          }
          frame #2 {
            # "Take an image"
            n260 = local read "Current Image Index"() -> (w462:i16)
            n261 = local read "Image Array"() -> (w465:T2[])
            n262 = local read "Camera Session"() -> (w469:T1)
            n263 = Increment(x=w462) -> (x+1=w461:i16)
            n264 = Index Array(array=w465, index=w462) -> (element=w468:T2)
            n265 = local write "Current Image Index"(w461) -> ()
            n266 = call <vilib>:"IMAQdx Snap2.vi"("error in"=w467, "Image In"=w468, "Session In"=w469) -> ("error out"=w466:errorcluster, "Image Out"=w464:T2, "Session Out"=w470:T1)  [unwired: 6 in]
            n267 = local write "error"(w466) -> ()
            n268 = local write "Camera Session"(w470) -> ()
            n269 = Replace Array Subset(array=w465, new element=w464, index=w462) -> (w463:T2[])
            n270 = local write "Image Array"(w463) -> ()
          }
        }
      }
    }
  }
